vi "test.ingest_journalJson.vi"   [LabVIEW 2020]
uses:
  datasources/source/create_s3.vi
  datasources/source/source.lvclass
  datasources/target/create_new.vi
  datasources/target/target.lvclass
  datasources/dataset/dataset.lvclass
  81c5314d-0c17-4e40-9591-806fc92e59be.vi
  Nominal Client/Nominal Client.lvclass
  40e2c779-94f0-4ff6-913c-6196809b7e71.vi
  Nominal Client/ingest_journalJson.vi
  datasources/source/create_gcs.vi
  datasources/target/create_from_existing.vi
  nominal types/channelConfig/channelConfig.lvclass
  nominal types/properties/properties.lvclass
  datasources/s3/s3.lvclass
  C:/code/labview-client/lv_src/Nominal Client/datasources/source/source.lvclass
  C:/code/labview-client/lv_src/Nominal Client/datasources/payload/payload.lvclass
  C:/code/labview-client/lv_src/Nominal Client/datasources/s3/s3.lvclass
  datasources/gcs/gcs.lvclass
  C:/code/labview-client/lv_src/Nominal Client/datasources/gcs/gcs.lvclass
types:
  T1 = cluster{"dataset":refnum<class "dataset.lvclass">, "channelConfig":refnum<class "channelConfig.lvclass">}
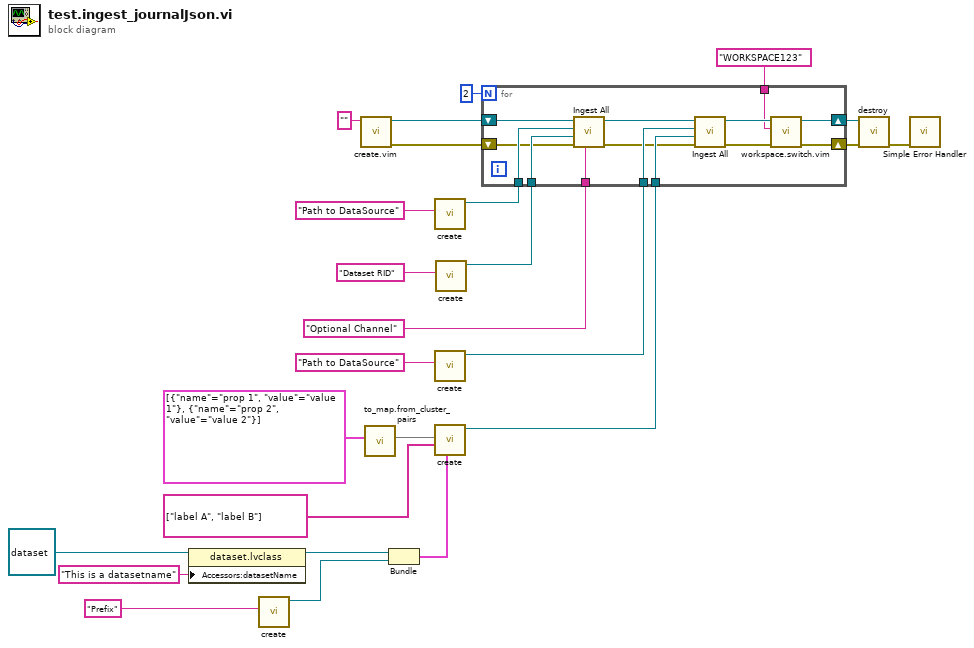
[diagram p0: block diagram]
diagram:
  n1 = property class="dataset.lvclass"(reference=refnum<class "dataset.lvclass"> refnum ("dataset"), "Accessors:datasetName"="This is a datasetname" ("datasetName")) -> (reference out=w16:refnum<class "dataset.lvclass">)  [unwired: 1 in, 1 out]
  n2 = call "create.vi"("prefixTreeDelimiter"="Prefix") -> ("channelConfig"=w5:refnum<class "channelConfig.lvclass">)  [unwired: 10 in]
  n3 = call "create.vim"("API Token (string or path)"="") -> ("error out"=w20:errorcluster, "Nominal Client"=w21:refnum<class "Nominal Client.lvclass">)  [unwired: 9 in]
  n4 = call "to_map.from_cluster_pairs.vi"("properties (cluster pairs)"=cluster{"name":string, "value":string}[] [{"name"="prop 1", "value"="value 1"}, {"name"="prop 2", "value"="value 2"}] ("properties")) -> ("properties (map)"=w2:map{string, string})  [unwired: 10 in]
  n5 = Bundle("dataset"=w16, "channelConfig"=w5) -> (w15:T1)  [unwired: 1 in]
  n6 = call-poly "create.vi"("Path"="Path to DataSource") -> ("source"=w7:refnum<class "s3.lvclass">)  [unwired: 10 in]
  n7 = call-poly "create.vi"("Path"="Path to DataSource") -> ("source"=w11:refnum<class "gcs.lvclass">)  [unwired: 10 in]
  n8 = call-poly "create.vi"("Optional"=w15, "Labels"=string[] ["label A", "label B"] ("labels"), "Properties"=w2) -> ("New Target"=w25:refnum<class "target.lvclass">)  [unwired: 8 in]
  n9 = call-poly "create.vi"("dataset RID"="Dataset RID" ("RID")) -> ("Existing Target"=w9:refnum<class "target.lvclass">)  [unwired: 10 in]
  n10 = for {
    N: 2 -> [_]
    tunnel: w9 -> [w39]
    tunnel: w7 -> [w38]
    tunnel: w11 -> [w37]
    tunnel: w25 -> [w36]
    shift-right: [w29] -> w22
    shift-left: w20 -> [w33]
    shift-right: [w28] -> w24
    shift-left: w21 -> [w32]
    tunnel: "WORKSPACE123" ("RID") -> [w27]
    tunnel: "Optional Channel" ("topic") -> [w26]
    n11 = call-poly "Ingest All.vi"("channel"=w26, "error in"=w33, "Target"=w39, "Source"=w38, "Nominal Client in"=w32) -> ("error out"=w34:errorcluster, "Nominal Client out"=w35:refnum<class "Nominal Client.lvclass">)  [unwired: 3 in, 2 out]
    n12 = call-poly "Ingest All.vi"("error in"=w34, "Target"=w36, "Source"=w37, "Nominal Client in"=w35) -> ("error out"=w30:errorcluster, "Nominal Client out"=w31:refnum<class "Nominal Client.lvclass">)  [unwired: 4 in, 2 out]
    n13 = call "workspace.switch.vim"("error in"=w30, "Workspace RID (string or path)"=w27, "Nominal Client in"=w31) -> ("error out"=w29:errorcluster, "Nominal Client out"=w28:refnum<class "Nominal Client.lvclass">)  [unwired: 7 in]
  }
  n14 = call "destroy.vi"("error in"=w22, "Nominal Client"=w24) -> ("error out"=w4:errorcluster)  [unwired: 9 in]
  n15 = call <vilib>:"Simple Error Handler.vi"("error in (no error)"=w4) -> ()  [unwired: 4 in, 5 out]
